vi "ParseLeidenComputerNames.vi"(8 "error in (no error)":errorcluster, 10 "AVS type":T1(ring) caption="Bridge Type", 11 "computer name":string="custardpie") -> (0 "error out":errorcluster, 2 "AVS Type":T2(ring)=enum."CF_Z_Bridge", 3 "FP Type":enum32{"CF", "Wet"}(ring))   [LabVIEW 2013]
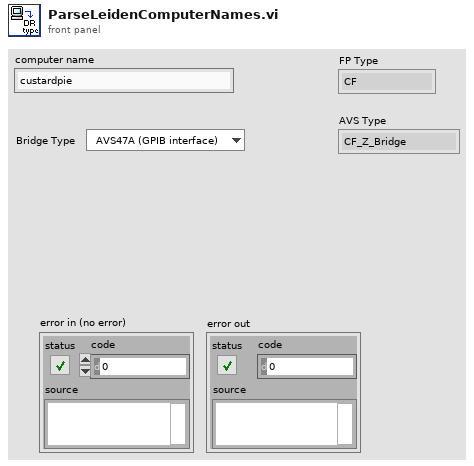
[diagram p1: front panel]
types:
  T1 = enum16{"AVS47A (GPIB interface)", "AVS47B (RS232 interface)", "AVS48", "AVS Emulation", "Impedance Bridge", "Disabled"}
  T2 = enum16{"CF", "CF_Z_Bridge", "MNK", "MNK_Z_Bridge"}
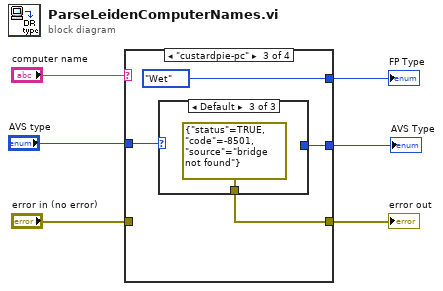
[diagram p0: block diagram]
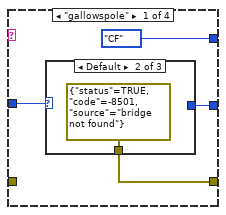
[diagram p2: hidden frame]
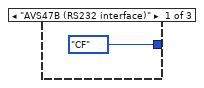
[diagram p3: hidden frame]
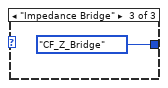
[diagram p4: hidden frame]
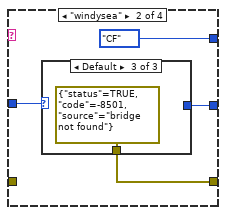
[diagram p5: hidden frame]
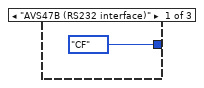
[diagram p6: hidden frame]
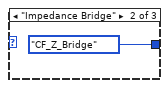
[diagram p7: hidden frame]
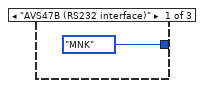
[diagram p8: hidden frame]
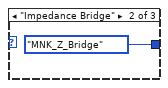
[diagram p9: hidden frame]
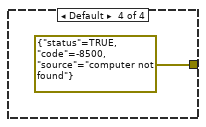
[diagram p10: hidden frame]
diagram:
  n1 = case shown="\"custardpie-pc\"" "computer name" {
    tunnel: [enum32{"CF", "Wet"}."CF" ("Type") enum32{"CF", "Wet"}."CF" ("Type") enum32{"CF", "Wet"}."Wet" ("Type") _] -> w6
    tunnel: "error in (no error)" -> [_ _ _ _]
    tunnel: [w7 w14 w21 errorcluster {"status"=TRUE, "code"=-8500, "source"="computer not found"} ("error in (no error)")] -> w3
    tunnel: "AVS type" -> [w9 w15 w22 _]
    tunnel: [w8 w16 w23 _] -> w1
    frame "gallowspole" {
      n2 = case shown="Default" w9 {
        tunnel: [T2."CF" ("AVS Type") _ T2."CF_Z_Bridge" ("AVS Type")] -> w8
        tunnel: [_ errorcluster {"status"=TRUE, "code"=-8501, "source"="bridge not found"} ("error in (no error)") _] -> w7
        frame "AVS47B (RS232 interface)" {
        }
        frame Default {
        }
        frame "Impedance Bridge" {
        }
      }
    }
    frame "windysea" {
      n3 = case shown="Default" w15 {
        tunnel: [T2."CF" ("AVS Type") T2."CF_Z_Bridge" ("AVS Type") _] -> w16
        tunnel: [_ _ errorcluster {"status"=TRUE, "code"=-8501, "source"="bridge not found"} ("error in (no error)")] -> w14
        frame "AVS47B (RS232 interface)" {
        }
        frame "Impedance Bridge" {
        }
        frame Default {
        }
      }
    }
    frame "custardpie-pc" {
      n4 = case shown="Default" w22 {
        tunnel: [T2."MNK" ("AVS Type") T2."MNK_Z_Bridge" ("AVS Type") _] -> w23
        tunnel: [_ _ errorcluster {"status"=TRUE, "code"=-8501, "source"="bridge not found"} ("error in (no error)")] -> w21
        frame "AVS47B (RS232 interface)" {
        }
        frame "Impedance Bridge" {
        }
        frame Default {
        }
      }
    }
    frame Default {
    }
  }
  "FP Type" <- w6
  "error out" <- w3
  "AVS Type" <- w1
